vi "DateTimeStringToSecond.vi"(10 "input string":string) -> (2 "time stamp":timestamp)   [LabVIEW 2012]
uses:
  <vilib>/Utility/miscctls.llb/LVDateTimeRec.ctl
panel:
  in  "date time rec":T1
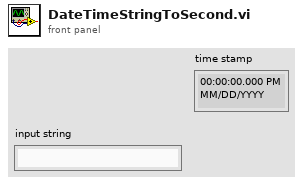
[diagram p1: front panel]
types:
  T1 = typedef "LVDateTimeRec.ctl" = cluster{"fractional second":dbl, "second":i32, "minute":i32, "hour":i32, "day of month":i32, "month":i32, "year":i32, "day of week":i32, "day of year":i32, "DST":i32}
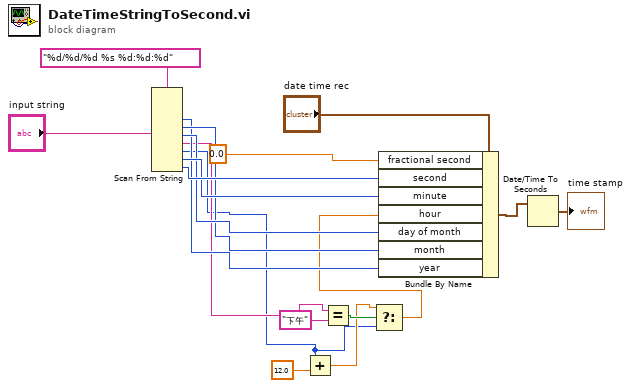
[diagram p0: block diagram]
diagram:
  n1 = Scan From String(format string="%d/%d/%d %s %d:%d:%d", input string="input string") -> (output 1=w11:i32, output 2=w12:i32, output 3=w13:i32, output 4=w6:string, output 5=w3:i32, output 6=w14:i32, output 7=w15:i32)  [unwired: 9 in, 3 out]
  n2 = Add(x=w3, y=12.0) -> (x+y=w7:dbl)
  n3 = Equal?(x=w6, y="下午") -> (x = y?=w9:bool)
  n4 = Select(t=w7, s=w9, f=w3) -> (s? t:f=w2:dbl)
  n5 = Bundle By Name(cluster="date time rec", "fractional second"=0.0, "second"=w15, "minute"=w14, "hour"=w2, "day of month"=w13, "month"=w12, "year"=w11) -> (w5:T1)
  n6 = Date/Time To Seconds(2:w5) -> (0:→"time stamp":timestamp)  [unwired: 1 in]
